vi "5 x Lesen CAN Konfig.vi"(5 "Datenfluss (in)":bool, 8 "Fehler (Eingang, kein Fehler)":errorcluster, 9 "Factorysettings":path, 11 "appended path":path) -> (0 "Fehler (Ausgang)":errorcluster, 3 "Konfig Daten 2":T1={"Baude Rate"=250000, "COM state"=144, "Frame-ID FTIR Start"=0, "Frame-ID FTIR End"=0, "Frame-ID Status Start"=0, "Frame-ID Status End"=0, "Zustand Information"=0, "Aktion"=0, "Frame-ID FTIR Arry"=[], "Frame-ID Status Arry"=[], "GPS Start"=0, "Interface"="CAN1"} {"Baude Rate" items=["40 kBaud"=40000, "50 kBaud"=50000, "62,5 kBaud"=62500, "80 kBaud"=80000, "83,3 kBaud"=83300, "100 kBaud"=100000, "125 kBaud"=125000, "160 kBaud"=160000, "200 kBaud"=200000, "250 kBaud"=250000, "400 kBaud"=400000, "500 kBaud"=500000, "800 kBaud"=800000, "1 MBaud"=1000000]}, 4 "Datenfluss (out)":bool)   [LabVIEW 2020, in "Konfig-Dateien.lvlib"]
uses:
  Konfig-Dateien.lvlib
  Seiten/CAN Konfig/Konfig Daten PC.ctl
  CAN Interface/Baude Rate.ctl
  SysLog/SysLog Interface cRIO.ctl
  SysLog/SysLog_cRIO.lvlib
  CAN Interface/CAN Interface.lvlib
  Seiten/CAN Konfig/CAN Konfig.lvlib
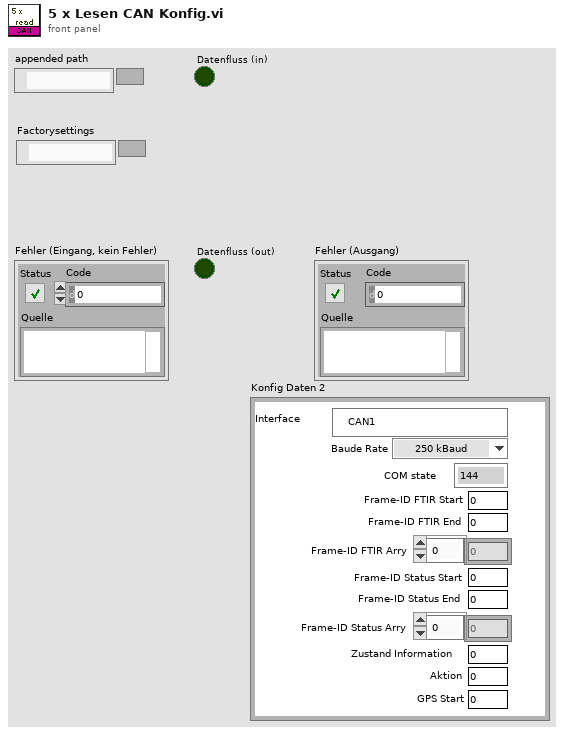
[diagram p1: front panel]
types:
  T1 = typedef "CAN Konfig.lvlib/Konfig Daten PC.ctl" = cluster{"Baude Rate":T2, "COM state":u8, "Frame-ID FTIR Start":u32, "Frame-ID FTIR End":u32, "Frame-ID Status Start":u32, "Frame-ID Status End":u32, "Zustand Information":u32, "Aktion":u32, "Frame-ID FTIR Arry":u32[], "Frame-ID Status Arry":u32[], "GPS Start":u32, "Interface":refnum<k21>}
  T2 = typedef "CAN Interface.lvlib/Baude Rate.ctl" = u32
  T3 = typedef "SysLog_cRIO.lvlib/SysLog Interface cRIO.ctl" = cluster{"FehlermeldungsCode":i32, "ErfolgsmeldungsCode":i32, "ParameterListenString":string, "intern":bool}
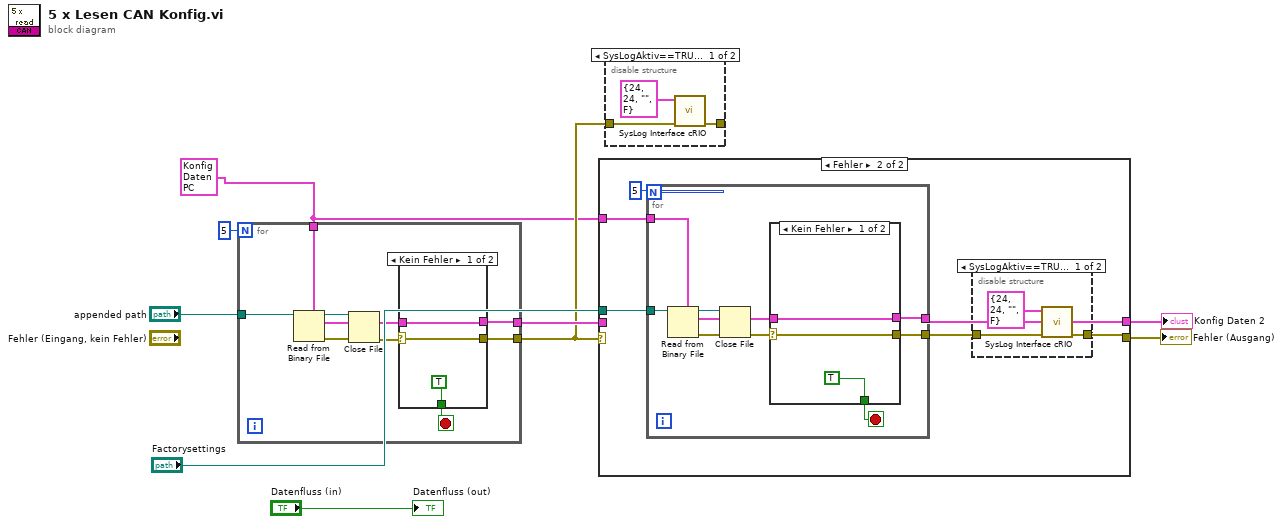
[diagram p0: block diagram]
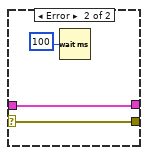
[diagram p5: hidden frame]
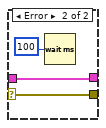
[diagram p6: hidden frame]
diagram:
  w2 = T1 {"Baude Rate"=250000, "COM state"=144, "Frame-ID FTIR Start"=0, "Frame-ID FTIR End"=0, "Frame-ID Status Start"=0, "Frame-ID Status End"=0, "Zustand Information"=0, "Aktion"=0, "Frame-ID FTIR Arry"=[], "Frame-ID Status Arry"=[], "GPS Start"=0, "Interface"="CAN1"} ("Konfig Daten 2")
  n1 = for {
    N: 5 -> [_]
    tunnel: [w15] -> w6
    tunnel: "appended path" -> [w18]
    tunnel: w2 -> [w11]
    tunnel: [w10] -> w3
    stop <- w17 stop-if-true
    n2 = Read from Binary File(5:w11, 11:w18) -> (0:w13:errorcluster, 2:w16:T1, 3:w14:refnum<file>)  [unwired: 4 in, 1 out]
    n3 = Close File(refnum=w14, error in=w13) -> (error out=w12:errorcluster)  [unwired: 1 out]
    n4 = case shown="Kein Fehler" w12 {
      selector: w12 -> [w20 w23]
      tunnel: [TRUE _] -> w17
      tunnel: [w19 w24] -> w15
      tunnel: w16 -> [w19 w24]
      tunnel: [w20 w23] -> w10
      frame No Error {
      }
      frame Error {
        n5 = Wait (ms)(milliseconds to wait=u32 100 ("Zu wartende ms")) -> ()  [unwired: 1 out]
      }
    }
  }
  n6 = case shown="Fehler" w3 {
    selector: w3 -> [w26 _]
    tunnel: w6 -> [w25 _]
    tunnel: "Factorysettings" -> [_ w31]
    tunnel: [w26 w29] -> w4
    tunnel: [w25 w28] -> w1
    tunnel: w2 -> [_ w27]
    frame No Error {
    }
    frame Error {
      n7 = for {
        N: 5 -> [_]
        tunnel: [w42] -> w28
        tunnel: w31 -> [w45]
        tunnel: [w38] -> w30
        tunnel: w27 -> [w37]
        stop <- w44 stop-if-true
        n8 = Read from Binary File(5:w37, 11:w45) -> (0:w41:errorcluster, 2:w43:T1, 3:w39:refnum<file>)  [unwired: 4 in, 1 out]
        n9 = Close File(refnum=w39, error in=w41) -> (error out=w40:errorcluster)  [unwired: 1 out]
        n10 = case shown="Kein Fehler" w40 {
          selector: w40 -> [w46 w50]
          tunnel: [TRUE _] -> w44
          tunnel: [w47 w51] -> w42
          tunnel: w43 -> [w47 w51]
          tunnel: [w46 w50] -> w38
          frame No Error {
          }
          frame Error {
            n11 = Wait (ms)(milliseconds to wait=u32 100 ("Zu wartende ms")) -> ()  [unwired: 1 out]
          }
        }
      }
      n12 = disable-structure shown="SysLogAktiv==TRUE" {
        disable-tunnel: w30 -> [w33 w36]
        disable-tunnel: [w34 w36] -> w29
        frame condition #0 (active) {
          n13 = call "SysLog Interface cRIO.vi"("Fehler (in)"=w33, "Cluster (in)"=T3 {"FehlermeldungsCode"=24, "ErfolgsmeldungsCode"=24, "ParameterListenString"="", "intern"=FALSE}) -> ("Fehler (Ausgang)"=w34:errorcluster)  [unwired: 9 in]
        }
        frame condition #1 {
        }
      }
    }
  }
  "Fehler (Ausgang)" <- w4
  "Konfig Daten 2" <- w1
  n14 = disable-structure shown="SysLogAktiv==TRUE" {
    disable-tunnel: w3 -> [w52 w55]
    disable-tunnel: [w53 w55] -> _
    frame condition #0 (active) {
      n15 = call "SysLog Interface cRIO.vi"("Fehler (in)"=w52, "Cluster (in)"=T3 {"FehlermeldungsCode"=24, "ErfolgsmeldungsCode"=24, "ParameterListenString"="", "intern"=FALSE}) -> ("Fehler (Ausgang)"=w53:errorcluster)  [unwired: 9 in]
    }
    frame condition #1 {
    }
  }
  "Datenfluss (out)" <- "Datenfluss (in)"
